vi "receive_data.vi"(0 "存盘":bool, 5 "error in (no error)":errorcluster, 9 "file path (dialog if empty)":path=path "E:/测试数据/新芯片") -> (4 "timeout?":bool, 6 "error out":errorcluster)   [LabVIEW 2016, in "BT-Android_interface.lvlib"]
uses:
  BT-Android_interface.lvlib
  mode.ctl
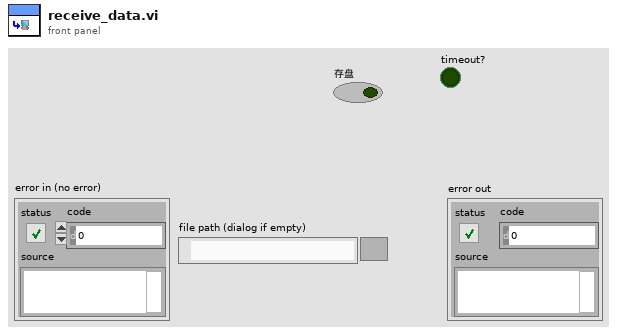
[diagram p1: front panel]
types:
  T1 = typedef "BT-Android_interface.lvlib/mode.ctl" = enum16{"init", "broadcast_data", "receive_data", "close"}
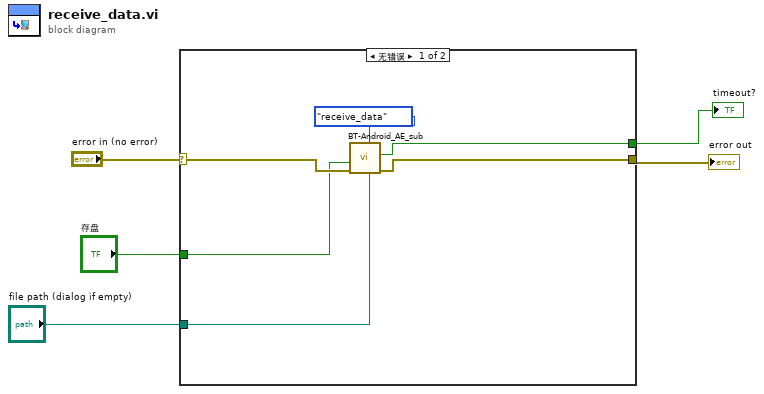
[diagram p0: block diagram]
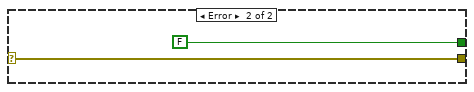
[diagram p2: hidden frame]
diagram:
  n1 = case shown="无错误" "error in (no error)" {
    selector: "error in (no error)" -> [w11 w13]
    tunnel: [w10 w13] -> w4
    tunnel: [w9 FALSE ("timeout?")] -> w3
    tunnel: "存盘" -> [w7 _]
    tunnel: "file path (dialog if empty)" -> [w6 _]
    frame No Error {
      n2 = call "BT-Android_AE_sub.vi"("file path (dialog if empty)"=w6, "mode"=mode."receive_data", "error in (no error)"=w11, "存盘"=w7) -> ("error IO"=w10:errorcluster, "timeout?"=w9:bool)  [unwired: 6 in]
    }
    frame Error {
    }
  }
  "error out" <- w4
  "timeout?" <- w3
